vi "API.vi"   [LabVIEW 2021]
uses:
  Msgs/Actor Create/Actor Create/Actor Create.lvclass
  Msgs/Actor Create/Actor Create Msg Strategy/Actor Create Msg Strategy.lvclass
  jettl/jettl.lvlib
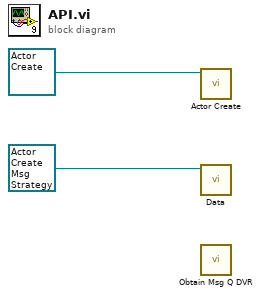
[diagram p0: block diagram]
diagram:
  n1 = call-dynamic "Actor Create.vi"("Actor Create in"=refnum<class "Actor Create.lvclass"> refnum ("Actor Create.lvlib:Actor Create.lvclass")) -> ()  [unwired: 10 in, 1 out]
  n2 = call "Data.vi"("Actor Create Msg Strategy in"=refnum<class "Actor Create Msg Strategy.lvclass"> refnum ("Actor Create.lvlib:Actor Create Msg Strategy.lvclass")) -> ()  [unwired: 9 in, 2 out]
  n3 = call "Obtain Msg Q DVR.vi"() -> ()  [unwired: 10 in, 2 out]
